vi "Text Viewer.vi"(8 "error in":errorcluster, 10 "Change Log Display":string) -> (0 "error out":errorcluster)   [LabVIEW 2023]
panel:
  in  "OK Button":bool
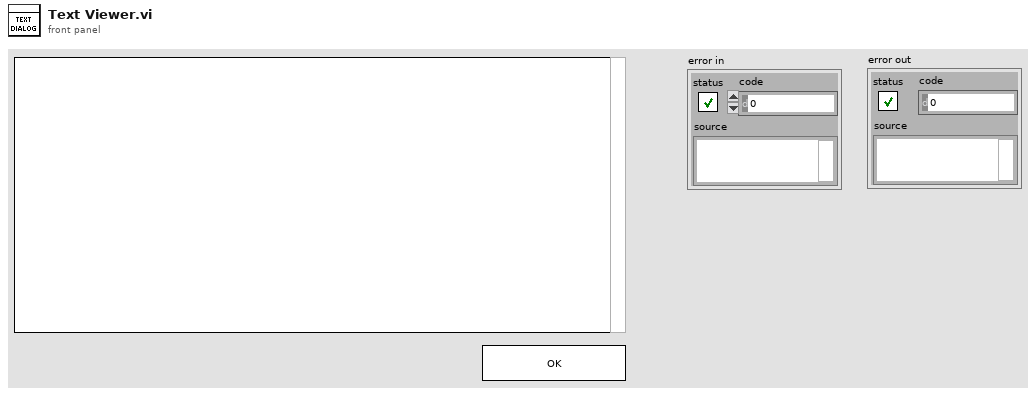
[diagram p1: front panel]
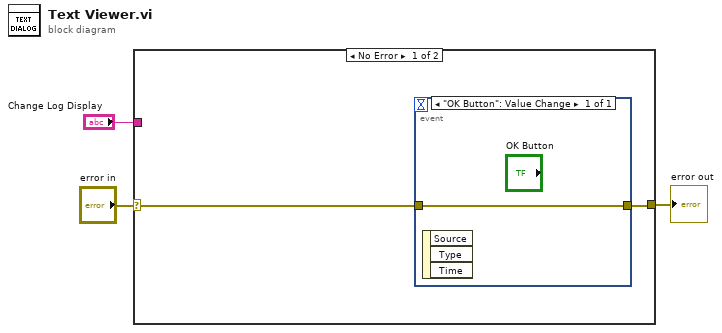
[diagram p0: block diagram]
diagram:
  n1 = case shown="No Error" "error in" {
    selector: "error in" -> [w4 w7]
    tunnel: [w5 w7] -> w2
    tunnel: "Change Log Display" -> [_ _]
    frame No Error {
      n2 = event shown="[0] \"OK Button\": Value Change" {
        selector: _ -> [_]
        dyn-events: _ -> [_]
        timeout: _ -> [_]
        tunnel: w4 -> [w6]
        tunnel: [w6] -> w5
        event "OK Button": Value Change {
          n3 = event-data() -> ()  [unwired: 1 in, 3 out]
        }
      }
    }
    frame Error {
    }
  }
  "error out" <- w2
